vi "Untitled 2.vi"() -> ()   [LabVIEW 2018]
panel:
  out "Boolean":bool
  in  "test":bool
  out "Time":u32
  out "Numeric 2":i32
  out "Numeric":i32
  out "relative seconds 2":dbl format="%_19f"
  in  "stop":bool
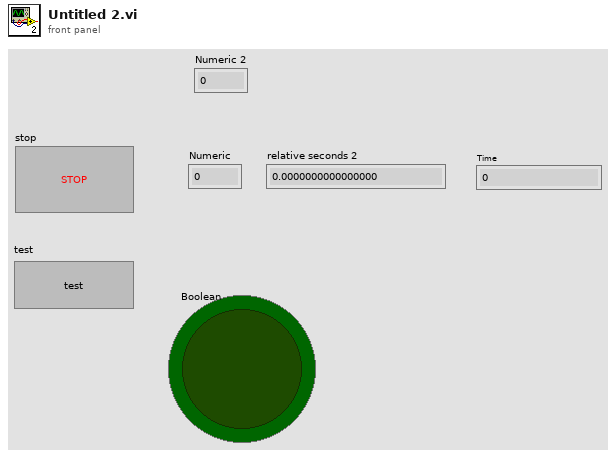
[diagram p1: front panel]
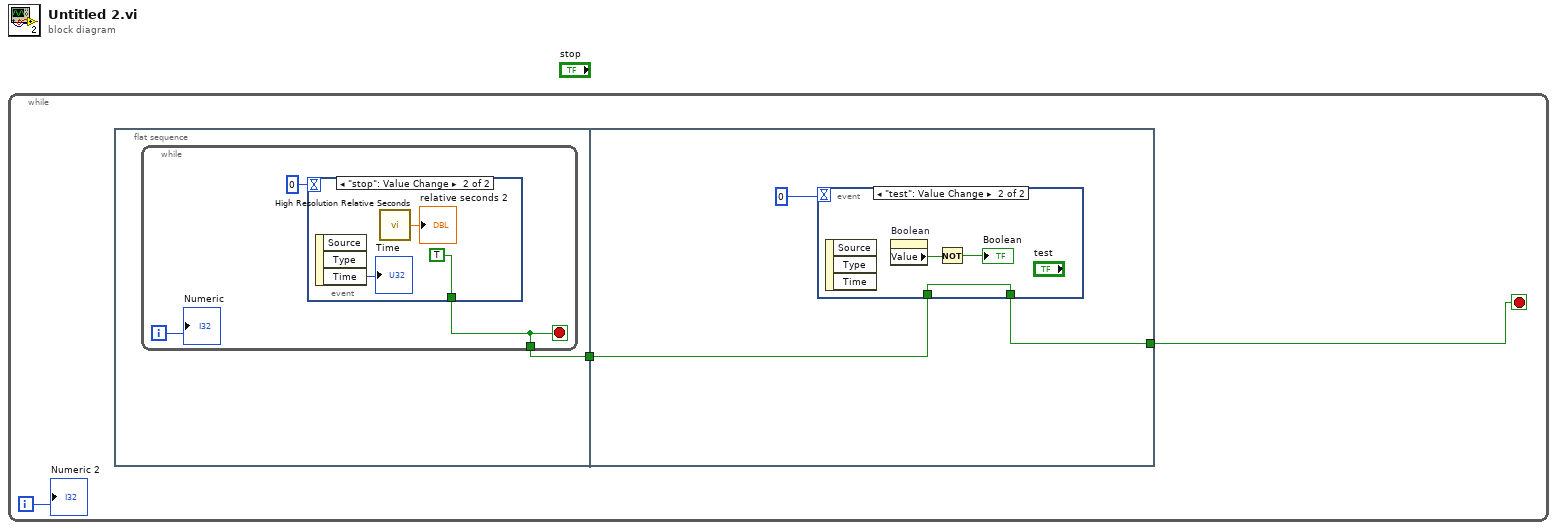
[diagram p0: block diagram]
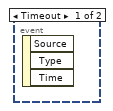
[diagram p2: hidden frame]
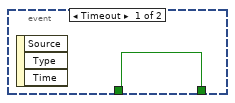
[diagram p3: hidden frame]
diagram:
  n1 = while {
    i -> [w3]
    stop <- w1 stop-if-true
    n2 = flat-sequence {
      tunnel: [w4] -> w2
      tunnel: w2 -> [w12]
      tunnel: [w11] -> w1
      frame #0 {
        n3 = while {
          tunnel: [w5] -> w4
          i -> [w6]
          stop <- w5 stop-if-true
          n4 = event shown="[1] \"stop\": Value Change" {
            selector: _ -> [_ _]
            dyn-events: _ -> [_ _]
            timeout: 0 -> [_ _]
            tunnel: [_ TRUE] -> w5
            event Timeout {
              n5 = event-data() -> ()  [unwired: 1 in, 3 out]
            }
            event "stop": Value Change {
              n6 = event-data() -> ("Time"=→"Time":u32)  [unwired: 1 in, 2 out]
              n7 = call <vilib>:"High Resolution Relative Seconds.vi"() -> ("relative seconds"=→"relative seconds 2":dbl)
            }
          }
          "Numeric" <- w6
        }
      }
      frame #1 {
        n8 = event shown="[1] \"test\": Value Change" {
          selector: _ -> [_ _]
          dyn-events: _ -> [_ _]
          timeout: 0 -> [_ _]
          tunnel: w12 -> [w14 w15]
          tunnel: [w14 w15] -> w11
          event Timeout {
            n9 = event-data() -> ()  [unwired: 1 in, 3 out]
          }
          event "test": Value Change {
            n10 = event-data() -> ()  [unwired: 1 in, 3 out]
            n11 = property on="Boolean" class="Bool (strict)"() -> ("Value"=w17:bool)  [unwired: 2 in, 2 out]
            n12 = Not(x=w17) -> (.not. x?=→"Boolean":bool)
          }
        }
      }
    }
    "Numeric 2" <- w3
  }
